vi "DemoGUI_XY.vi"() -> ()   [LabVIEW 2015]
uses:
  C:/LabNation/SmartScopeApp/SmartScope/bin/Windows/AnyCPU/Debug/LabNation.DeviceInterface.dll
  SmartScopeApp/SmartScope/bin/Windows/AnyCPU/Debug/LabNation.DeviceInterface.dll
panel:
  out "XY Graph":T1(graph)
  in  "ChB Offset":dbl(slide)=2.0 scale=-4.0..4.0
  in  "ChB V/div":i8(knob)=5 caption="Knob" scale=0.0..7.0
  in  "TriggerHoldoff":dbl(slide) scale=-0.0005..0.0005
  in  "Time/div":i8(knob)=6 caption="Knob" scale=0.0..12.0
  in  "ChA Offset":dbl(slide) scale=-4.0..4.0
  in  "ChA V/div":i8(knob)=5 caption="Knob" scale=0.0..7.0
  in  "TriggerLevel":dbl(slide) scale=-2.612244897959184..5.387755102040816 scale format="%#_6f"
  out "Waveform Graph":dbl[][](graph)
  out "Connected":bool
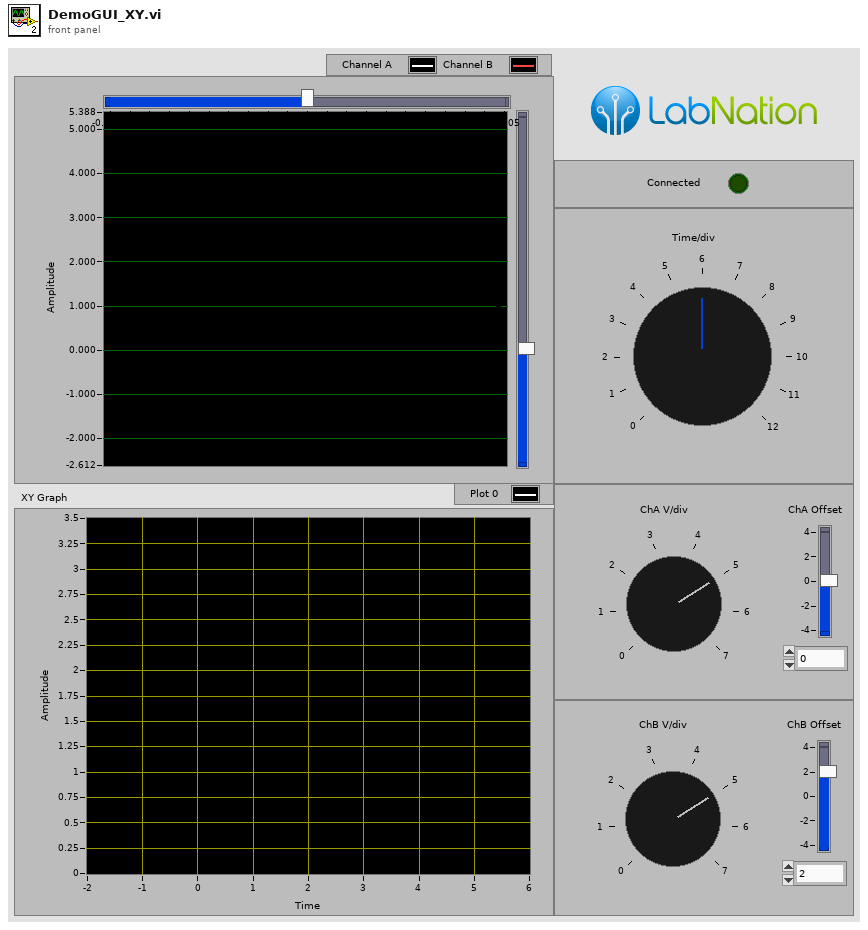
[diagram p1: front panel]
types:
  T1 = cluster{"Waveform Graph":dbl[], "Waveform Graph":dbl[]}
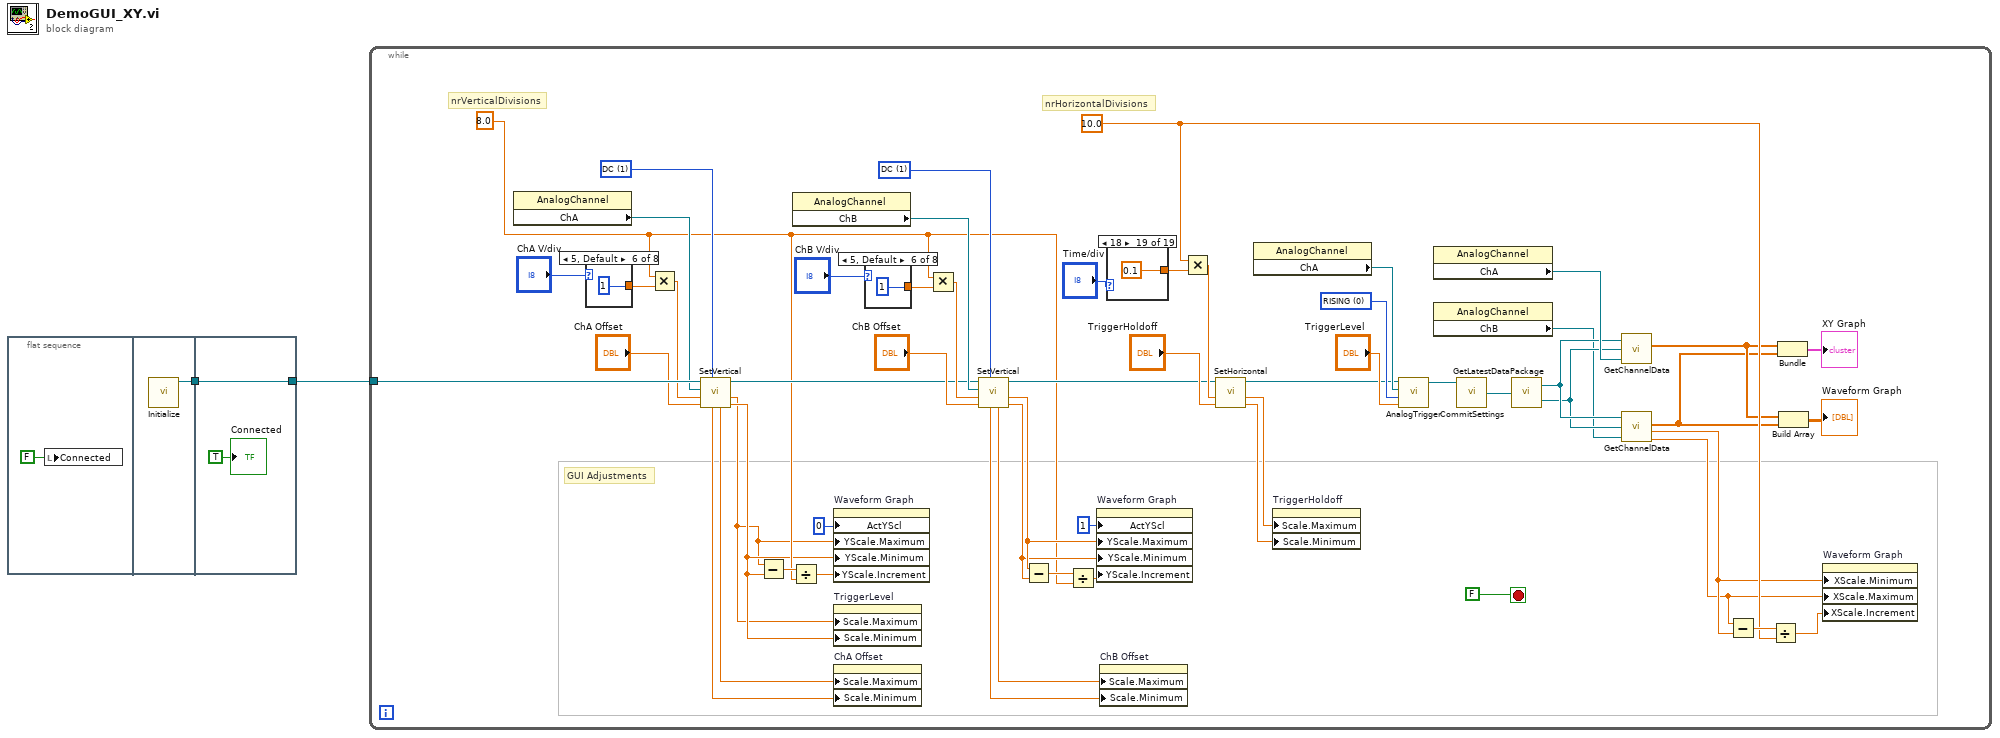
[diagram p0: block diagram]
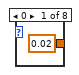
[diagram p2: hidden frame]
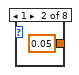
[diagram p3: hidden frame]
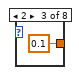
[diagram p4: hidden frame]
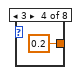
[diagram p5: hidden frame]
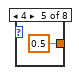
[diagram p6: hidden frame]
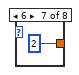
[diagram p7: hidden frame]
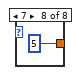
[diagram p8: hidden frame]
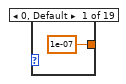
[diagram p9: hidden frame]
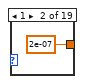
[diagram p10: hidden frame]
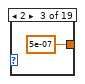
[diagram p11: hidden frame]
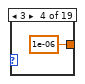
[diagram p12: hidden frame]
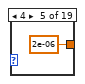
[diagram p13: hidden frame]
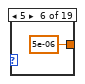
[diagram p14: hidden frame]
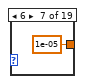
[diagram p15: hidden frame]
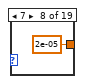
[diagram p16: hidden frame]
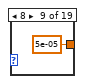
[diagram p17: hidden frame]
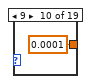
[diagram p18: hidden frame]
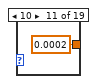
[diagram p19: hidden frame]
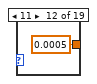
[diagram p20: hidden frame]
diagram:
  n1 = flat-sequence {
    tunnel: [w4] -> w1
    tunnel: [w6] -> w2
    tunnel: w1 -> [w6]
    frame #0 {
      n2 = local write "Connected"(FALSE ("Connected")) -> ()
    }
    frame #1 {
      n3 = call "Initialize.vi"() -> ("SmartScope out"=w4:refnum<k24>)  [unwired: 1 in]
    }
    frame #2 {
      "Connected" <- TRUE ("Connected")
    }
  }
  n4 = while {
    tunnel: w2 -> [w59]
    stop <- FALSE stop-if-true
    w33 = 1 items=["AC", "DC"] ("coupling")
    w42 = 0 items=["RISING", "FALLING", "ANY"] ("edge")
    w46 = 1 items=["AC", "DC"] ("coupling")
    w38 = 10.0 ("y")
    w24 = 8.0 ("y")
    # "GUI Adjustments"
    # "nrHorizontalDivisions"
    # "nrVerticalDivisions"
    n5 = property class="AnalogChannel"() -> ("ChA"=w54:refnum<k24>)  [unwired: 2 in, 2 out]
    n6 = case shown="5, Default" "ChA V/div" {
      tunnel: [0.02 0.05 0.1 0.2 0.5 1 2 5] -> w45
      frame 0 {
      }
      frame 1 {
      }
      frame 2 {
      }
      frame 3 {
      }
      frame 4 {
      }
      frame 5, Default {
      }
      frame 6 {
      }
      frame 7 {
      }
    }
    n7 = Multiply(x=w24, y=w45) -> (x*y=w56:dbl)
    n8 = call "SetVertical.vi"("coupling"=w46, "Offset"="ChA Offset", "Range"=w56, "AnalogChannel"=w54, "SmartScope in"=w59) -> ("GraphMin"=w21:dbl, "GraphMax"=w20:dbl, "SmartScope out"=w31:refnum<k24>, "OffsetMax"=w58:dbl, "OffsetMin"=w57:dbl)  [unwired: 2 in]
    n9 = Subtract(x=w20, y=w21) -> (x-y=w47:dbl)
    n10 = Divide(x=w47, y=w24) -> (x/y=w22:dbl)
    n11 = property class="AnalogChannel"() -> ("ChB"=w34:refnum<k24>)  [unwired: 2 in, 2 out]
    n12 = property on="Waveform Graph" class="WFGraph (strict)"("ActYScl"=0 ("Active Y Scale"), "YScale.Maximum"=w20, "YScale.Minimum"=w21, "YScale.Increment"=w22) -> ()  [unwired: 2 in, 2 out]
    n13 = property on="TriggerLevel" class="Slide (strict)"("Scale.Maximum"=w20, "Scale.Minimum"=w21) -> ()  [unwired: 2 in, 2 out]
    n14 = property on="ChA Offset" class="Slide (strict)"("Scale.Maximum"=w58, "Scale.Minimum"=w57) -> ()  [unwired: 2 in, 2 out]
    n15 = case shown="5, Default" "ChB V/div" {
      tunnel: [0.02 0.05 0.1 0.2 0.5 1 2 5] -> w32
      frame 0 {
      }
      frame 1 {
      }
      frame 2 {
      }
      frame 3 {
      }
      frame 4 {
      }
      frame 5, Default {
      }
      frame 6 {
      }
      frame 7 {
      }
    }
    n16 = Multiply(x=w24, y=w32) -> (x*y=w36:dbl)
    n17 = call "SetVertical.vi"("coupling"=w33, "Offset"="ChB Offset", "Range"=w36, "AnalogChannel"=w34, "SmartScope in"=w31) -> ("GraphMin"=w26:dbl, "GraphMax"=w27:dbl, "SmartScope out"=w30:refnum<k24>, "OffsetMax"=w18:dbl, "OffsetMin"=w17:dbl)  [unwired: 2 in]
    n18 = Subtract(x=w27, y=w26) -> (x-y=w25:dbl)
    n19 = Divide(x=w25, y=w24) -> (x/y=w23:dbl)
    n20 = property on="Waveform Graph" class="WFGraph (strict)"("ActYScl"=u32 1 ("Plot.Y Scale Index"), "YScale.Maximum"=w27, "YScale.Minimum"=w26, "YScale.Increment"=w23) -> ()  [unwired: 2 in, 2 out]
    n21 = property on="ChB Offset" class="Slide (strict)"("Scale.Maximum"=w18, "Scale.Minimum"=w17) -> ()  [unwired: 2 in, 2 out]
    n22 = case shown="18" "Time/div" {
      tunnel: [1e-07 2e-07 5e-07 1e-06 2e-06 5e-06 1e-05 2e-05 5e-05 0.0001 0.0002 0.0005 0.001 0.002 0.005 0.01 0.02 0.05 0.1] -> w44
      frame 0, Default {
      }
      frame 1 {
      }
      frame 2 {
      }
      frame 3 {
      }
      frame 4 {
      }
      frame 5 {
      }
      frame 6 {
      }
      frame 7 {
      }
      frame 8 {
      }
      frame 9 {
      }
      frame 10 {
      }
      frame 11 {
      }
      frame 12 {
      }
      frame 13 {
      }
      frame 14 {
      }
      frame 15 {
      }
      frame 16 {
      }
      frame 17 {
      }
      frame 18 {
      }
    }
    n23 = Multiply(x=w38, y=w44) -> (x*y=w50:dbl)
    n24 = call "SetHorizontal.vi"("TriggerHoldoff"="TriggerHoldoff", "ViewportLength"=w50, "SmartScope in"=w30) -> ("TrigSliderMin"=w51:dbl, "TrigSliderMax"=w52:dbl, "SmartScope out"=w40:refnum<k24>)  [unwired: 2 in]
    n25 = property class="AnalogChannel"() -> ("ChA"=w43:refnum<k24>)  [unwired: 2 in, 2 out]
    n26 = property on="TriggerHoldoff" class="Slide (strict)"("Scale.Maximum"=w52, "Scale.Minimum"=w51) -> ()  [unwired: 2 in, 2 out]
    n27 = call "AnalogTrigger.vi"("EdgeType"="TriggerLevel", "TriggerLevel"=w42, "AnalogChannel"=w43, "SmartScope in"=w40) -> ("SmartScope out"=w39:refnum<k24>)
    n28 = property class="AnalogChannel"() -> ("ChA"=w15:refnum<k24>)  [unwired: 2 in, 2 out]
    n29 = property class="AnalogChannel"() -> ("ChB"=w12:refnum<k24>)  [unwired: 2 in, 2 out]
    n30 = call "CommitSettings.vi"("SmartScope in"=w39) -> ("SmartScope out"=w16:refnum<k24>)
    n31 = call "GetLatestDataPackage.vi"("SmartScope in"=w16) -> ("SmartScope out"=w14:refnum<k24>, "DataPackage"=w13:refnum<k24>)
    n32 = call "GetChannelData.vi"("SmartScope in"=w14, "LatestDataPackage"=w13, "AnalogChannel"=w15) -> ("Waveform Graph"=w9:dbl[])  [unwired: 3 out]
    n33 = call "GetChannelData.vi"("SmartScope in"=w14, "LatestDataPackage"=w13, "AnalogChannel"=w12) -> ("Waveform Graph"=w8:dbl[], "ViewportBegin"=w11:dbl, "ViewportEnd"=w10:dbl)  [unwired: 1 out]
    n34 = Subtract(x=w10, y=w11) -> (x-y=w49:dbl)
    n35 = Divide(x=w49, y=w38) -> (x/y=w48:dbl)
    n36 = Bundle("Waveform Graph"=w9, "Waveform Graph"=w8) -> (→"XY Graph":T1)  [unwired: 1 in]
    n37 = Build Array(w9, w8) -> (→"Waveform Graph":dbl[][])
    n38 = property on="Waveform Graph" class="WFGraph (strict)"("XScale.Minimum"=w11, "XScale.Maximum"=w10, "XScale.Increment"=w48) -> ()  [unwired: 2 in, 2 out]
  }
